vi "首页显示设置.vi"() -> ()   [LabVIEW 2016]
uses:
  <vilib>/Utility/config.llb/NI_LVConfig.lvlib
panel:
  in  "首页显示信息设置":T1={"水温"=FALSE, "pH"=FALSE, "DO"=FALSE, "Cond"=FALSE, "Turb"=FALSE, "氨氮"=FALSE, "总磷"=FALSE, "总氮"=FALSE, "CODMn"=FALSE, "CODCr"=FALSE, "水位"=FALSE, "流速"=FALSE, "瞬时流量"=FALSE, "室温"=TRUE, "湿度"=TRUE, "叶绿素a"=FALSE, "藻密度"=FALSE}
  in  "关闭":bool
  # "首页显示信息设置"
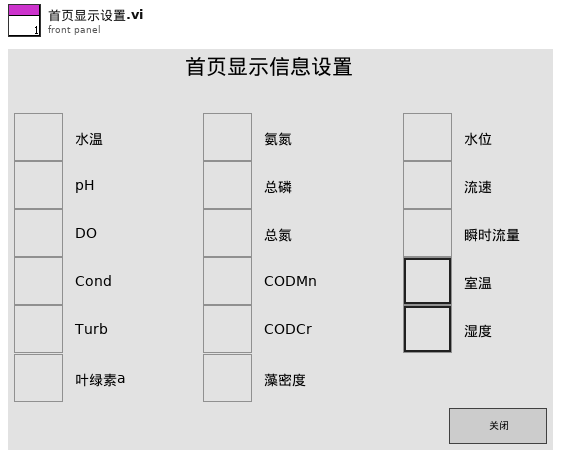
[diagram p1: front panel]
types:
  T1 = cluster{"水温":bool, "pH":bool, "DO":bool, "Cond":bool, "Turb":bool, "氨氮":bool, "总磷":bool, "总氮":bool, "CODMn":bool, "CODCr":bool, "水位":bool, "流速":bool, "瞬时流量":bool, "室温":bool, "湿度":bool, "叶绿素a":bool, "藻密度":bool}
  T2 = typedef "NI_LVConfig.lvlib/Config Data RefNum.ctl" = refnum<k1>
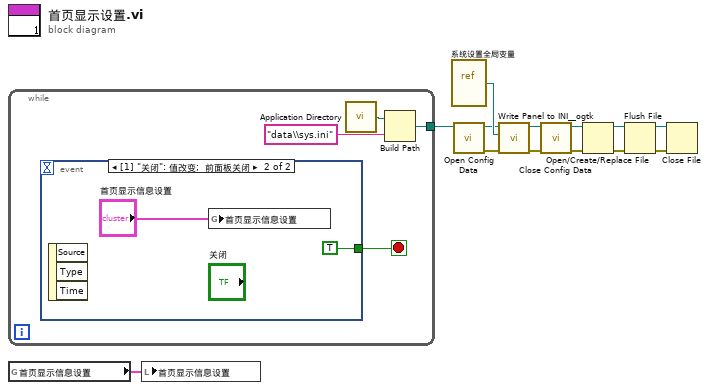
[diagram p0: block diagram]
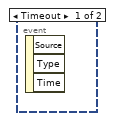
[diagram p2: hidden frame]
diagram:
  n1 = while {
    tunnel: [w14] -> w7
    stop <- w17 stop-if-true
    n2 = event shown="[1] \"关闭\": 值改变;  前面板关闭" {
      selector: _ -> [_ _]
      dyn-events: _ -> [_ _]
      timeout: _ -> [_ _]
      tunnel: [_ TRUE] -> w17
      event Timeout {
        n3 = event-data() -> ()  [unwired: 1 in, 3 out]
      }
      event "关闭": Value Change; Panel Close {
        n4 = event-data() -> ()  [unwired: 1 in, 3 out]
        n5 = global write "系统设置全局变量.vi" "首页显示信息设置"("首页显示信息设置") -> ()
      }
    }
    n6 = call <vilib>:"Application Directory.vi"() -> ("Application Directory"=w15:path)
    n7 = Build Path(base path=w15, name or relative path="data\\sys.ini" ("名称或相对路径")) -> (appended path=w14:path)
  }
  n8 = global read "系统设置全局变量.vi" "首页显示信息设置"() -> (w8:T1)
  n9 = local write "首页显示信息设置"(w8) -> ()
  n10 = vi-ref "系统设置全局变量.vi"() -> (w10:refnum<vi>)
  n11 = call <vilib>:"Open Config Data.vi"("configuration file path"=w7) -> ("error out"=w12:errorcluster, "refnum"=w9:T2)  [unwired: 8 in, 1 out]
  n12 = call <userlib>:"Write Panel to INI__ogtk.vi"("error in (no error)"=w12, "VI ref"=w10, "refnum"=w9) -> ("error out"=w13:errorcluster, "refnum out"=w11:T2)  [unwired: 7 in]
  n13 = call <vilib>:"Close Config Data.vi"("error in (no error)"=w13, "refnum"=w11) -> ("error out"=w1:errorcluster, "file path"=w2:path)  [unwired: 8 in]
  n14 = Open/Create/Replace File(file path (use dialog)=w2, error in=w1) -> (refnum out=w5:refnum<file>, error out=w6:errorcluster)  [unwired: 4 in, 1 out]
  n15 = Flush File(refnum=w5, error in=w6) -> (refnum out=w4:refnum<file>, error out=w3:errorcluster)
  n16 = Close File(refnum=w4, error in=w3) -> ()  [unwired: 2 out]
